vi "AC-Transfer_mod2.vi"() -> ()   [LabVIEW 2014]
uses:
  <vilib>/Analysis/4window.llb/windowTd.ctl
  <vilib>/Analysis/1siggen.llb/Ramp Pattern by Samples.vi
  <vilib>/DAQmx/create/channels.llb/DAQmx Create Channel (AI-Voltage-Basic).vi
  <vilib>/DAQmx/create/channels.llb/DAQmx Create Channel (AO-Voltage-Basic).vi
  <vilib>/DAQmx/configure/timing.llb/DAQmx Timing (Sample Clock).vi
  <vilib>/DAQmx/configure/trigger.llb/DAQmx Start Trigger (Digital Edge).vi
  <vilib>/DAQmx/write.llb/DAQmx Write (Analog Wfm 1Chan NSamp).vi
  <vilib>/DAQmx/read.llb/DAQmx Read (Analog 2D DBL NChan NSamp).vi
  <vilib>/measure/maspectr.llb/FFT Power Spectrum and PSD for 1 Chan.vi
  <vilib>/measure/maspectr.llb/Frequency Response Function (Mag-Phase) 1-1.vi
  <resource>/objmgr/daqmx.rc
  <vilib>/measure/NI_MABase.lvlib
  <vilib>/Analysis/NI_AALBase.lvlib
  <vilib>/measure/NI_MAPro.lvlib
  <vilib>/Analysis/NI_AALPro.lvlib
panel:
  out "Phase response":cluster{dbl[], dbl[]}(graph)
  out "Magnitude response":cluster{dbl[], dbl[]}(graph)
  in  "Sweep poins":i32=30
  in  "Sweep end [Hz]":dbl=1000.0
  in  "Sweep start [Hz]":dbl=1.0
  in  "Amplitude":dbl=1.0
  out "Actual Fs [Hz]":dbl
  in  "Sampling freq [Hz]":dbl=100000.0 format="%#_6p"
  in  "Sampled points":i32=65536
  in  "Trigger Source (ai/StartTrigger)":tag="/cDAQ2/ai/StartTrigger"
  in  "Output Channel (Mod2/ao1)":tag="cDAQ2Mod2/ao0"
  in  "Input Channels (Mod1/ai0:1)":tag="cDAQ2Mod1/ai0:1"
  # "Channel Settings"
  # "Measurement settings"
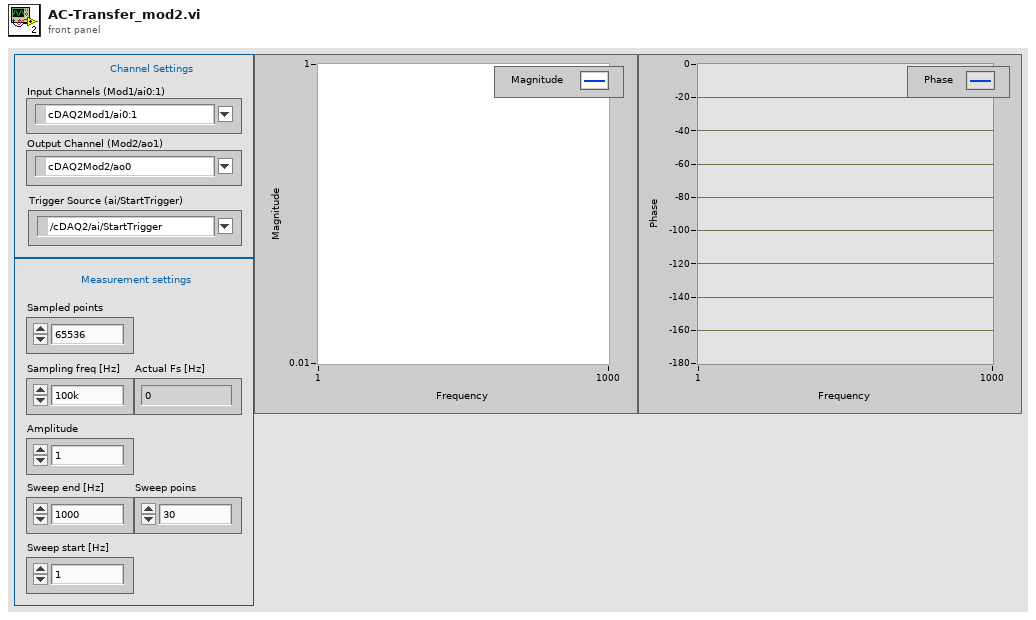
[diagram p1: front panel]
types:
  T1 = typedef "NI_AALPro.lvlib/windowTd.ctl" = u32
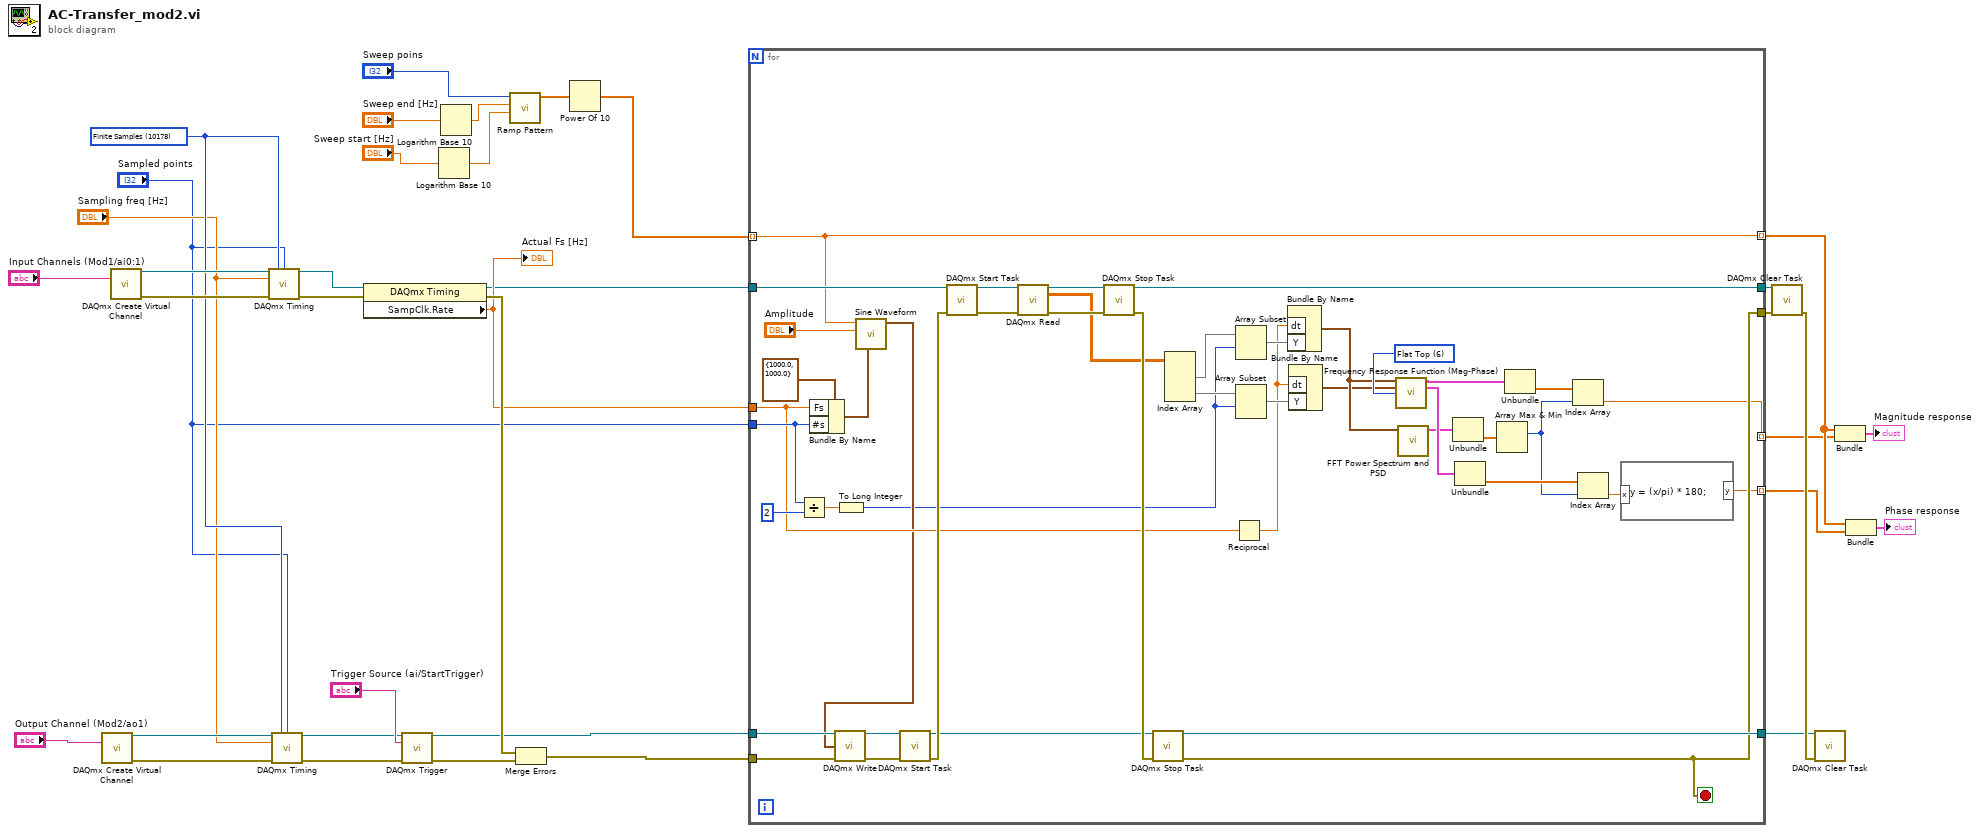
[diagram p0: block diagram]
diagram:
  w29 = 10178 items=["Finite Samples"=10178, "Continuous Samples"=10123, "Hardware Timed Single Point"=12522] ("sample mode")
  n1 = call-poly <vilib>:"DAQmx Create Virtual Channel.vi"("physical channels"="Output Channel (Mod2/ao1)") -> ("task out"=w35:refnum<k21>, "error out"=w33:errorcluster)  [unwired: 13 in]
  n2 = call-poly <vilib>:"DAQmx Create Virtual Channel.vi"("physical channels"="Input Channels (Mod1/ai0:1)") -> ("task out"=w36:refnum<k21>, "error out"=w34:errorcluster)  [unwired: 13 in]
  n3 = call-poly <vilib>:"DAQmx Timing.vi"("task/channels in"=w36, "sample mode"=w29, "samples per channel"="Sampled points", "rate"="Sampling freq [Hz]", "error in"=w34) -> ("task out"=w32:refnum<k21>, "error out"=w31:errorcluster)  [unwired: 9 in]
  n4 = call-poly <vilib>:"DAQmx Timing.vi"("task/channels in"=w35, "sample mode"=w29, "samples per channel"="Sampled points", "rate"="Sampling freq [Hz]", "error in"=w33) -> ("task out"=w4:refnum<k21>, "error out"=w30:errorcluster)  [unwired: 9 in]
  n5 = property class="DAQmx Timing"(reference=w32, error in=w31) -> (reference out=w17:refnum<k21>, error out=w25:errorcluster, "SampClk.Rate"=w22:dbl)
  "Actual Fs [Hz]" <- w22
  n6 = call-poly <vilib>:"DAQmx Trigger.vi"("task/channels in"=w4, "source"="Trigger Source (ai/StartTrigger)", "error in"=w30) -> ("task out"=w18:refnum<k21>, "error out"=w24:errorcluster)  [unwired: 11 in]
  n7 = Logarithm Base 10(1:"Sweep start [Hz]") -> (0:w6:dbl)
  n8 = Logarithm Base 10(1:"Sweep end [Hz]") -> (0:w8:dbl)
  n9 = call-poly <vilib>:"Ramp Pattern.vi"("start"=w6, "end"=w8, "samples"="Sweep poins") -> ("Ramp Pattern"=w10:dbl[])  [unwired: 7 in, 1 out]
  n10 = Merge Errors(w25, w24) -> (w19:errorcluster)
  n11 = Power Of 10(x=w10) -> (10^x=w9:dbl[])
  n12 = for {
    tunnel: w22 -> [w54]
    tunnel: "Sampled points" -> [w59]
    tunnel: w9 -> [w42] mode=indexing
    tunnel: w19 -> [w76]
    tunnel: w18 -> [w75]
    tunnel: w17 -> [w70]
    tunnel: [w63] -> w15
    tunnel: [w67] -> w16
    tunnel: [w64] -> w13
    tunnel: [w45] -> w2 mode=indexing
    tunnel: [w37] -> w1 mode=indexing
    tunnel: [w42] -> w3 mode=indexing
    stop <- w63 stop-if-true
    w50 = T1 6 items=["Rectangle"=0, "Hanning"=1, "Hamming"=2, "Blackman-Harris"=3, "Exact Blackman"=4, "Blackman"=5, "Flat Top"=6, "4 Term B-Harris "=7, "7 Term B-Harris"=8, "Low Sidelobe"=9, "Blackman Nuttall"=11, "Triangle"=30, "Bartlett-Hanning"=31, "Bohman"=32, "Parzen"=33, "Welch"=34, "Kaiser"=60, "Dolph-Chebyshev"=61, "Gaussian"=62] ("window")
    n13 = Divide(x=w59, y=2) -> (x/y=w57:dbl)
    n14 = Bundle By Name(cluster=cluster{"Fs":dbl, "#s":dbl} {"Fs"=1000.0, "#s"=1000.0} ("sampling info"), "Fs"=w54, "#s"=w59) -> (w80:cluster{"Fs":dbl, "#s":dbl})
    n15 = To Long Integer(number=w57) -> (32bit integer=w40:i32)
    n16 = call <vilib>:"Sine Waveform.vi"("sampling info"=w80, "amplitude"="Amplitude", "frequency"=w42) -> ("signal out"=w41:waveform(dbl))  [unwired: 7 in, 1 out]
    n17 = call-poly <vilib>:"DAQmx Write.vi"("task/channels in"=w75, "data"=w41, "error in"=w76) -> ("task out"=w74:refnum<k21>, "error out"=w77:errorcluster)  [unwired: 10 in, 1 out]
    n18 = call <vilib>:"DAQmx Start Task.vi"("task/channels in"=w74, "error in"=w77) -> ("task out"=w65:refnum<k21>, "error out"=w71:errorcluster)  [unwired: 12 in]
    n19 = call <vilib>:"DAQmx Start Task.vi"("task/channels in"=w70, "error in"=w71) -> ("task out"=w73:refnum<k21>, "error out"=w72:errorcluster)  [unwired: 12 in]
    n20 = call-poly <vilib>:"DAQmx Read.vi"("task/channels in"=w73, "error in"=w72) -> ("task out"=w69:refnum<k21>, "data"=w62:dbl[][], "error out"=w68:errorcluster)  [unwired: 11 in]
    n21 = call <vilib>:"DAQmx Stop Task.vi"("task/channels in"=w69, "error in"=w68) -> ("task out"=w67:refnum<k21>, "error out"=w66:errorcluster)  [unwired: 12 in]
    n22 = call <vilib>:"DAQmx Stop Task.vi"("task/channels in"=w65, "error in"=w66) -> ("task out"=w64:refnum<k21>, "error out"=w63:errorcluster)  [unwired: 12 in]
    n23 = Index Array(array=w62) -> (element #1=w61:dbl[], element #2=w60:dbl[])  [unwired: 4 in]
    n24 = Reciprocal(x=w54) -> (1/x=w39:dbl)
    n25 = Array Subset(array=w61, index=w40) -> (w56:dbl[])  [unwired: 1 in]
    n26 = Array Subset(array=w60, index=w40) -> (w55:dbl[])  [unwired: 1 in]
    n27 = Bundle By Name("dt"=w39, "Y"=w56) -> (w44:waveform(dbl))  [unwired: 1 in]
    n28 = Bundle By Name("dt"=w39, "Y"=w55) -> (w43:waveform(dbl))  [unwired: 1 in]
    n29 = call-poly <vilib>:"Frequency Response Function (Mag-Phase).vi"("time signal X"=w44, "time signal Y"=w43, "window"=w50) -> ("magnitude"=w48:cluster{"f0":dbl, "df":dbl, "magnitude":dbl[]}, "phase"=w51:cluster{"f0":dbl, "df":dbl, "phase":dbl[]})  [unwired: 7 in, 4 out]
    n30 = call-poly <vilib>:"FFT Power Spectrum and PSD.vi"("time signal"=w44) -> ("Power Spectrum / PSD"=w49:cluster{"f0":dbl, "df":dbl, "magnitude":dbl[]})  [unwired: 7 in, 3 out]
    n31 = Unbundle(w49) -> ("magnitude"=w53:dbl[])  [unwired: 2 out]
    n32 = Unbundle(w51) -> ("phase"=w52:dbl[])  [unwired: 2 out]
    n33 = Array Max & Min(array=w53) -> (max index (indices)=w46:i32)  [unwired: 3 out]
    n34 = Unbundle(w48) -> ("magnitude"=w47:dbl[])  [unwired: 2 out]
    n35 = Index Array(array=w47, index=w46) -> (element=w45:dbl)
    n36 = Index Array(array=w52, index=w46) -> (element=w38:dbl)
    n37 = formula code="y = (x/pi) * 180;"("x"=w38) -> ("y"=w37:dbl)
  }
  n38 = call <vilib>:"DAQmx Clear Task.vi"("task in"=w16, "error in"=w15) -> ("error out"=w14:errorcluster)  [unwired: 13 in]
  n39 = call <vilib>:"DAQmx Clear Task.vi"("task in"=w13, "error in"=w14) -> ()  [unwired: 13 in, 1 out]
  n40 = Bundle(w3, w2) -> (→"Magnitude response":cluster{dbl[], dbl[]})  [unwired: 1 in]
  n41 = Bundle(w3, w1) -> (→"Phase response":cluster{dbl[], dbl[]})  [unwired: 1 in]
